vi "Create Counter Output PWM Module.vi"   [LabVIEW 2017, in "Scan Engine Scripting.lvlib"]
doc: "Creates and configures an instance of a counter output PWM module that can be used to set a slot in a scan engine custom device chassis."
uses:
  Scan Engine Scripting.lvlib
  NI 9474/NI 9474.lvclass
  NI 9475/NI 9475.lvclass
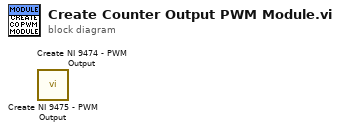
[diagram p0: block diagram]
diagram:
  n1 = call "Create NI 9475 - PWM Output.vi"() -> ()  [unwired: 10 in, 2 out]
  n2 = call "Create NI 9474 - PWM Output.vi"() -> ()  [unwired: 10 in, 2 out]
